vi "Collect 106E Data.vi"(0 "Reset Rain Closure":bool, 1 "Reset Forced Power Closure":bool, 2 "Boolean":bool, 4 "Remote Enable":bool, 5 "Close Slide Roof":bool, 6 "Rain Detector ON":bool, 7 "Open Slide Roof":bool, 8 "Boolean 2":bool, 9 "Boolean 3":bool, 10 "Close Drop Roof":bool, 11 "Mains/Battery":bool) -> (3 "String":string)   [LabVIEW 2009]
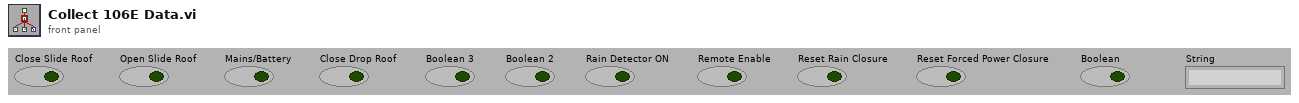
[diagram p1: front panel]
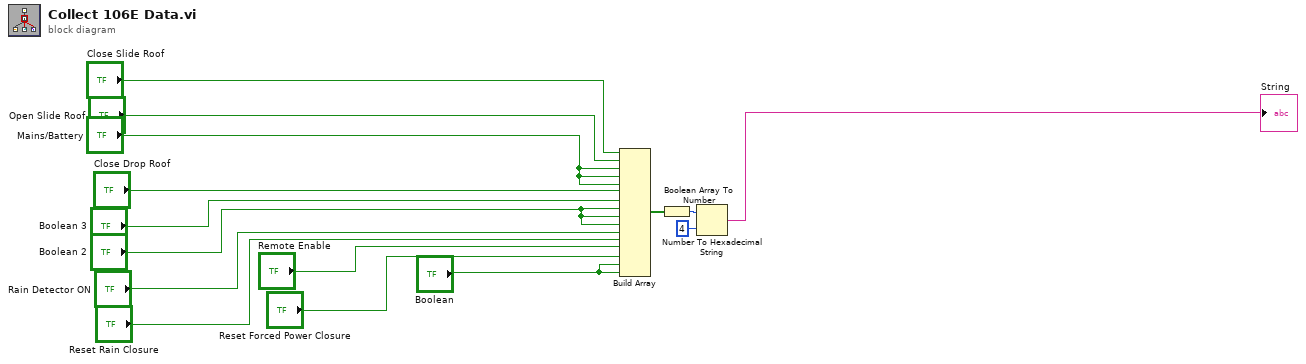
[diagram p0: block diagram]
diagram:
  n1 = Build Array("Close Slide Roof", "Open Slide Roof", "Mains/Battery", "Mains/Battery", "Mains/Battery", "Close Drop Roof", "Boolean 3", "Boolean 2", "Boolean 2", "Boolean 2", "Rain Detector ON", "Reset Rain Closure", "Remote Enable", "Reset Forced Power Closure", "Boolean", "Boolean") -> (w2:bool[])
  n2 = Boolean Array To Number(Boolean array=w2) -> (number=w3:u32)
  n3 = Number To Hexadecimal String(1:i16 4 ("width (-)"), 2:w3) -> (0:→"String":string)
